vi "SG_NetworkReceiver.vi"(8 "error in (no error)":errorcluster, 11 "Gserver in":refnum<class "Gserver.lvclass">) -> (0 "error out":errorcluster, 2 "RX":bool, 3 "Gserver out":refnum<class "Gserver.lvclass">)   [LabVIEW 2020, in "Sgraph_lib_V1.lvlib" / "Gserver.lvclass"]
doc: "Andre Koelewijn, 26 June 2023\n\nSgraph Network Receiver\nLoops over the list of connections and checks if there is new information to process.\nWhen info is received: then process it onto the Gserver Queue"
uses:
  Gserver.lvclass
  Gserver.lvclass/Gserver.ctl
  controls/Typedef_Gviewer-Query.ctl
  controls/Typedef_QueryType.ctl
  Builds/Sgraph_lib_V1.lvlib
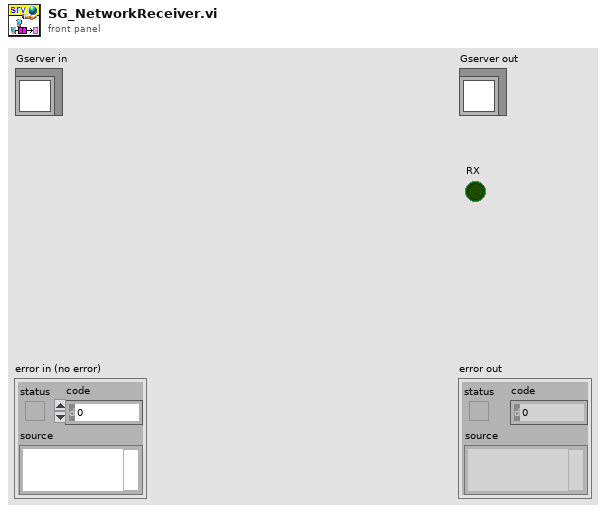
[diagram p1: front panel]
types:
  T1 = typedef "Sgraph_lib_V1.lvlib/Gserver.lvclass/Typedef_Gviewer-Query.ctl" = cluster{"Query_type":T2, "data":variant, "Source":string, "Time Stamp":timestamp}
  T2 = typedef "Sgraph_lib_V1.lvlib/Gserver.lvclass/Typedef_QueryType.ctl" = enum16{"Subscribe", "SubscribeNetw", "DataRequest", "RequestAllTags", "RequestIniPath", "FAMMstarted", "SetClientOptions", "GviewerUpdate", "OpenNewGraph", "CloseClient", "CloseAllClients", "Close Gserver", "OpenMemoryMap", "MeMapDataRequest", "MeMapDataResponse", "OpenDBeditor", "CheckDBeditorRunning", "StoppedDBeditor", "SaveDB_TAGpropRecord", "ConfirmDB_TAGpropSave", "GetXconstraints", "OpenNewNetworkGraph"}
  T3 = typedef "Sgraph_lib_V1.lvlib/Gserver.lvclass/Typedef_Sgraph_Query.ctl" = cluster{"ViewportName":string, "Tags":string[], "Time-Start":timestamp, "Time-End":timestamp, "Pixels":i32, "Live":T4, "TimeSpan(sec)":dbl, "GViewer-Queue":refnum<queue>, "Network":bool, "IP-address":string, "Port":u16, "connection-ID":refnum<k5>, "TCP-buffer":string}
  T4 = typedef "Sgraph_lib_V1.lvlib/Gviewer.lvclass/Typedef_Live.ctl" = enum16{"Live View", "Freeze"}
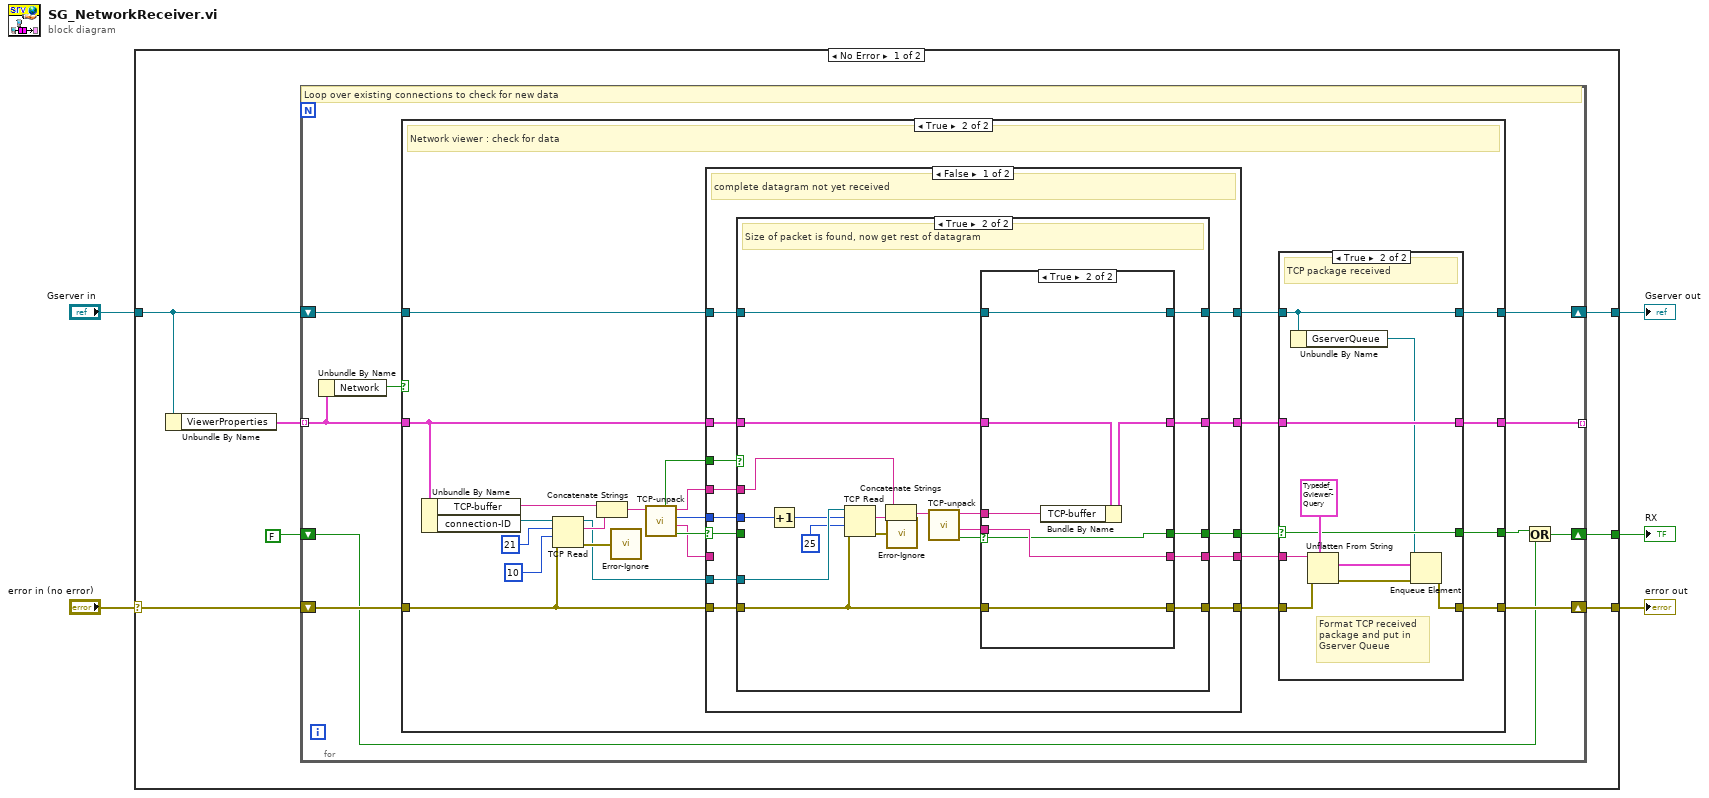
[diagram p0: block diagram]
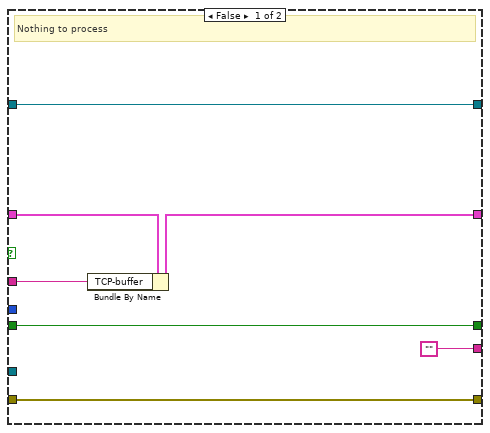
[diagram p4: hidden frame]
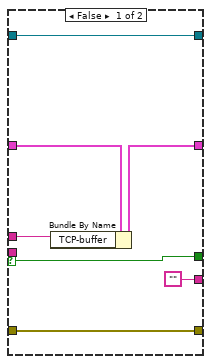
[diagram p5: hidden frame]
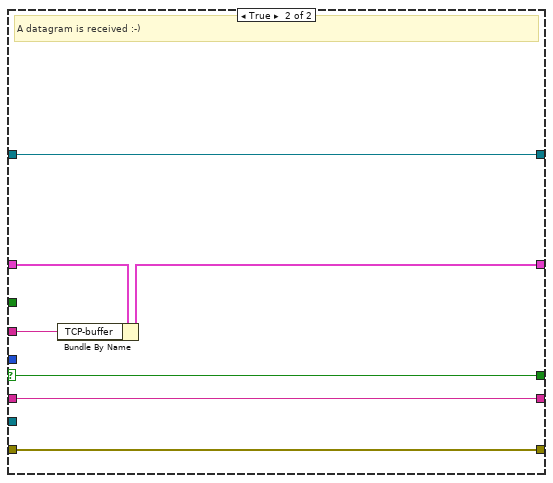
[diagram p6: hidden frame]
diagram:
  n1 = case shown="No Error" "error in (no error)" {
    selector: "error in (no error)" -> [w10 w127]
    tunnel: [w8 w127] -> w4
    tunnel: [w9 w126] -> w2
    tunnel: "Gserver in" -> [w11 w126]
    tunnel: [w6 _] -> w1
    frame No Error {
      n2 = Unbundle By Name(w11) -> ("ViewerProperties"=w12:T3[])
      n3 = for {
        tunnel: w12 -> [w17] mode=indexing
        shift-right: [w19] -> w9
        shift-left: w11 -> [w21]
        shift-right: [w18] -> w8
        shift-left: w10 -> [w20]
        tunnel: [w16] -> _ mode=indexing
        shift-right: [w13] -> w6
        shift-left: FALSE -> [w15]
        # "Loop over existing connections to check for new data"
        n4 = Unbundle By Name(w17) -> ("Network"=w22:bool)
        n5 = case shown="True" w22 {
          tunnel: w21 -> [w26 w47]
          tunnel: w20 -> [w25 w38]
          tunnel: [w26 w29] -> w19
          tunnel: [w25 w34] -> w18
          tunnel: w17 -> [w24 w40]
          tunnel: [w24 w27] -> w16
          tunnel: [FALSE w31] -> w14
          frame False {
            # "Queue viewer: no action needed here"
          }
          frame True {
            # "Network viewer : check for data"
            n6 = Unbundle By Name(w40) -> ("TCP-buffer"=w43:string, "connection-ID"=w51:refnum<k5>)
            n7 = TCP Read(connection ID=w51, bytes to read=21, error in (no error)=w38, 9:10 ("timeout ms (25000)")) -> (connection ID out=w36:refnum<k5>, data out=w42:string, error out=w37:errorcluster)  [unwired: 1 in]
            n8 = Concatenate Strings(w43, w42) -> (w41:string)
            n9 = call "Error-Ignore.vi"("error in"=w37) -> ()  [unwired: 9 in]
            n10 = call "TCP-unpack.vi"("TCP RX in"=w41) -> ("Success"=w48:bool, "TCP data"=w46:string, "bytecount"=w39:i32, "TCP RX out (rest)"=w45:string, "CountOK"=w44:bool)  [unwired: 6 in]
            n11 = case shown="False" w48 {
              selector: w48 -> [w67 w119]
              tunnel: w47 -> [w77 w124]
              tunnel: w38 -> [w75 w125]
              tunnel: [w76 w124] -> w30
              tunnel: [w74 w125] -> w33
              tunnel: w46 -> [_ w120]
              tunnel: w45 -> [w71 w123]
              tunnel: w44 -> [w78 _]
              tunnel: w40 -> [w73 w121]
              tunnel: [w72 w122] -> w28
              tunnel: w39 -> [w70 _]
              tunnel: w36 -> [w69 _]
              tunnel: [w68 w120] -> w35
              tunnel: [w66 w119] -> w32
              frame False {
                # "complete datagram not yet received"
                n12 = case shown="True" w78 {
                  tunnel: w77 -> [w85 w103]
                  tunnel: [w85 w101] -> w76
                  tunnel: w75 -> [w84 w104]
                  tunnel: [w84 w102] -> w74
                  tunnel: w73 -> [w83 w100]
                  tunnel: [w82 w99] -> w72
                  tunnel: w71 -> [w81 w97]
                  tunnel: w70 -> [_ w94]
                  tunnel: w69 -> [_ w98]
                  tunnel: ["" w96] -> w68
                  tunnel: w67 -> [w80 _]
                  tunnel: [w80 w95] -> w66
                  frame False {
                    # "Nothing to process"
                    n13 = Bundle By Name(cluster=w83, "TCP-buffer"=w81) -> (w82:T3)
                  }
                  frame True {
                    # "Size of packet is found, now get rest of datagram"
                    n14 = Increment(x=w94) -> (x+1=w86:i32)
                    n15 = TCP Read(connection ID=w98, bytes to read=w86, error in (no error)=w104, 9:25 ("timeout ms (25000)")) -> (data out=w92:string, error out=w87:errorcluster)  [unwired: 1 in, 1 out]
                    n16 = Concatenate Strings(w97, w92) -> (w91:string)
                    n17 = call "Error-Ignore.vi"("error in"=w87) -> ()  [unwired: 9 in]
                    n18 = call "TCP-unpack.vi"("TCP RX in"=w91) -> ("Success"=w90:bool, "TCP data"=w88:string, "TCP RX out (rest)"=w89:string)  [unwired: 6 in, 2 out]
                    n19 = case shown="True" w90 {
                      selector: w90 -> [w107 w112]
                      tunnel: w104 -> [w106 w118]
                      tunnel: [w106 w118] -> w102
                      tunnel: w103 -> [w108 w117]
                      tunnel: [w108 w117] -> w101
                      tunnel: w100 -> [w111 w115]
                      tunnel: w89 -> [w109 w116]
                      tunnel: [w110 w114] -> w99
                      tunnel: ["" w113] -> w96
                      tunnel: w88 -> [_ w113]
                      tunnel: [w107 w112] -> w95
                      frame False {
                        n20 = Bundle By Name(cluster=w111, "TCP-buffer"=w109) -> (w110:T3)
                      }
                      frame True {
                        n21 = Bundle By Name(cluster=w115, "TCP-buffer"=w116) -> (w114:T3)
                      }
                    }
                  }
                }
              }
              frame True {
                # "A datagram is received :-)"
                n22 = Bundle By Name(cluster=w121, "TCP-buffer"=w123) -> (w122:T3)
              }
            }
            n23 = case shown="True" w32 {
              selector: w32 -> [w54 w62]
              tunnel: w35 -> [_ w64]
              tunnel: [w55 w56] -> w34
              tunnel: w33 -> [w55 w63]
              tunnel: [w54 w62] -> w31
              tunnel: w30 -> [w53 w60]
              tunnel: [w53 w60] -> w29
              tunnel: w28 -> [w52 w61]
              tunnel: [w52 w61] -> w27
              frame False {
                # "not TCP data"
              }
              frame True {
                # "Format TCP received\npackage and put in\nGserver Queue"
                # "TCP package received"
                n24 = Unbundle By Name(w60) -> ("GserverQueue"=w59:refnum<queue>)
                n25 = Unflatten From String(type=T1 {"Query_type"=enum."Subscribe", "data"=variant, "Source"="", "Time Stamp"=timestamp(0 s since 1904-01-01)} ("element"), binary string=w64, error in (no error)=w63) -> (value=w57:T1, error out=w58:errorcluster)  [unwired: 2 in, 1 out]
                n26 = Enqueue Element(queue=w59, element=w57, error in (no error)=w58) -> (error out=w56:errorcluster)  [unwired: 1 in, 2 out]
              }
            }
          }
        }
        n27 = Or(x=w14, y=w15) -> (x .or. y?=w13:bool)
      }
    }
    frame Error {
    }
  }
  "error out" <- w4
  "Gserver out" <- w2
  "RX" <- w1
